vi "Communication.vi"() -> ()   [LabVIEW 2016, in "Hall Effect Library.lvlib"]
uses:
  Hall Effect Library.lvlib
  Public/Controls/Message Types.ctl
panel:
  out "KHEL Event":refnum<user-event>
  out "KHEL Msg Queue":refnum<queue>
  in  "KHEL Notifyer":refnum<notifier>
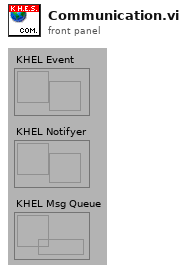
[diagram p1: front panel]
diagram:
